vi "getCalParam.vi"(3 "calType":enum16{"INTERNAL_CAL", "FULL_CAL"}(ring), 5 "Calibration Params":T1) -> (1 "value":dbl format="%.2f")   [LabVIEW 2012]
uses:
  Cal Parameters.ctl
  bin/OVA32.dll
panel:
  # "CAL_START_WL=0,       //start wavelength\n    CAL_RANGE_LENGTH,  //wavelength range length\n    CAL_NUM_AVGS,          //current num averages\n    CAL_RES,                     //current resolution\n    CAL_DECI,                   //current decimation factor\n    CAL_MEAS,                  //measurement type (0:Reflection  1:Transmission)\n    \n    //Limits\n    CAL_MIN_AVGS_ALLOWED,   //min # of avgs allowed for selected range\n    CAL_MAX_AVGS_ALLOWED,   //max # of avgs allowed for selected range\n    CAL_MIN_START_WL,       //min start wavelength of cal\n    CAL_CENTER,      //center wavelength of cal\n    CAL_END_WL,             //end wavelength (not a member of the structure)   \n    CAL_RANGE_WL,      //range(nm) of cal\n    CAL_RANGE_LENGTHS              //wavelength range lengths array"
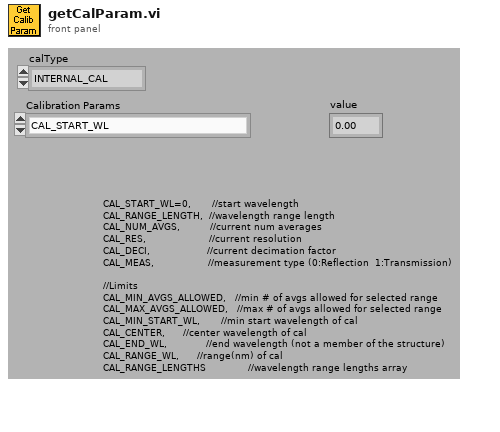
[diagram p1: front panel]
types:
  T1 = typedef "Cal Parameters.ctl" = enum16{"CAL_START_WL", "CAL_RANGE_LENGTH", "CAL_NUM_AVGS", "CAL_RES", "CAL_DECI", "CAL_MEAS", "CAL_MIN_AVGS", "CAL_MAX_AVGS", "CAL_MIN_START_WL", "CAL_CENTER_WL", "CAL_END_WL", "CAL_RANGE", "CAL_RANGE_LENGTHS"}
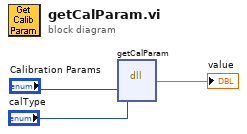
[diagram p0: block diagram]
diagram:
  n1 = dll-call lib="C:/_src/OVA5000_DSP_falcon/Software/LabVIEW/OVA/SDK/OVA_5000_SDK_v5.14.3/bin/OVA32.dll" fn="getCalParam"("param"="Calibration Params", "calType"="calType") -> (→"value":dbl)  [unwired: 5 in, 2 out]
